vi "ASCStringToRTUString.vi"(8 "CMDString":string) -> (0 "RTUString":string)   [LabVIEW 2023]
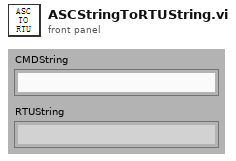
[diagram p1: front panel]
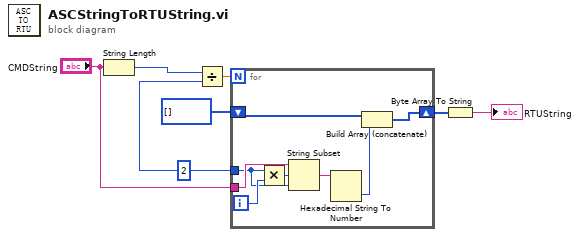
[diagram p0: block diagram]
diagram:
  w4 = 2
  n1 = String Length(string="CMDString") -> (length=w7:i32)
  n2 = Divide(x=w7, y=w4) -> (x/y=w6:dbl)
  n3 = for {
    N: w6 -> [_]
    tunnel: "CMDString" -> [w14]
    tunnel: w4 -> [w12]
    shift-right: [w8] -> w2
    shift-left: u32[] [] -> [w9]
    i -> [w15]
    n4 = Multiply(x=w12, y=w15) -> (x*y=w13:i32)
    n5 = String Subset(string=w14, offset (0)=w13, length (rest)=w12) -> (substring=w11:string)
    n6 = Hexadecimal String To Number(string=w11) -> (number=w10:u32)  [unwired: 2 in, 1 out]
    n7 = Build Array (concatenate)(w9, w10) -> (w8:u32[])
  }
  n8 = Byte Array To String(unsigned byte array=w2) -> (string=→"RTUString":string)
